vi "Actor Core.vi"(8 "error in":errorcluster, 11 "Chef Controller in":refnum<class "Chef Controller.lvclass">) -> (0 "error out":errorcluster, 3 "Actor out":refnum<class "Actor.lvclass">)   [LabVIEW 2024, in "Chef Controller.lvlib" / "Chef Controller.lvclass"]
doc: "<p>(<strong>Filename</strong>: <span class=\"dnl\">Actor Framework.lvlib:Actor.lvclass:Actor Core.vi</span>)</p>\n<p>Receives messages to the actor, reacts to them, and initiates any error handling that may shut the actor down.</p>\n<p>Descendant classes may override this VI to append parallel tasks for the actor to complete while it handles messages. Overrides use the <a href=\"nihelplauncher://docs/csh?context=lvcore_glang_udclass\">Call Parent Class Method</a> node.</p>"
uses:
  Chef Controller.lvclass
  Chef Controller.lvclass/Chef Controller.ctl
  <vilib>/ActorFramework/Actor/Actor.lvclass
  Chef View/Chef View.lvclass
  C:/Program Files/National Instruments/LabVIEW 2024/vi.lib/ActorFramework/Actor/Actor.lvclass
  G:/Leveling/LabVIEW/Learning/Actor Framework/chef/Chef View/Chef View.lvclass
  G:/Leveling/LabVIEW/Learning/Actor Framework/chef/Chef Controller/Chef Controller/Chef Controller.lvclass
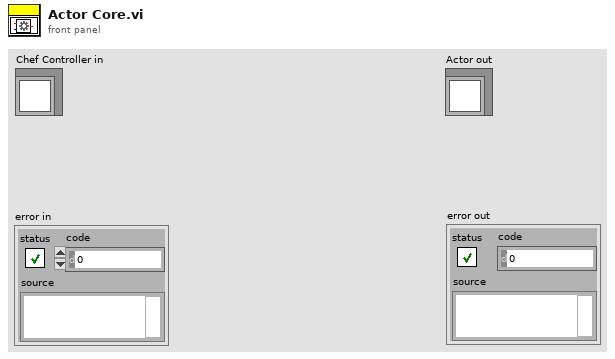
[diagram p1: front panel]
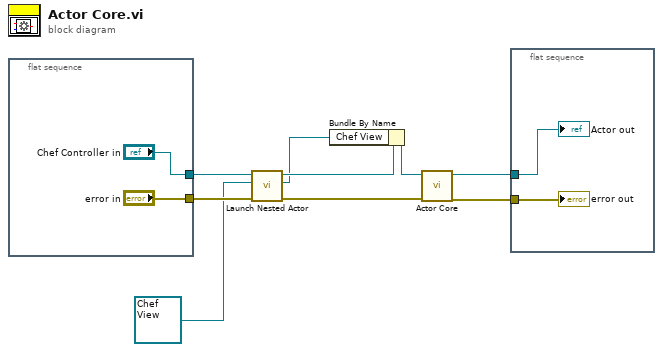
[diagram p0: block diagram]
diagram:
  n1 = flat-sequence {
    tunnel: ["error in"] -> w7
    tunnel: ["Chef Controller in"] -> w5
    frame #0 {
    }
  }
  n2 = call <vilib>:"Launch Nested Actor.vi"("error in (no error)"=w7, "Nested Actor"=refnum<class "Chef View.lvclass"> refnum ("Chef View.lvlib:Chef View.lvclass"), "Caller Actor in"=w5) -> ("error out"=w6:errorcluster, "Nested Actor's Enqueuer"=w1:refnum<class "Message Enqueuer.lvclass">, "Caller Actor out"=w4:refnum<class "Chef Controller.lvclass">)  [unwired: 6 in]
  n3 = Bundle By Name(cluster=w4, "Chef View"=w1) -> (w2:refnum<class "Chef Controller.lvclass">)
  n4 = call-parent "Actor Core.vi"("error in"=w6, "Actor in"=w2) -> ("error out"=w9:errorcluster, "Actor out"=w8:refnum<class "Actor.lvclass">)  [unwired: 8 in]
  n5 = flat-sequence {
    tunnel: w9 -> [w13]
    tunnel: w8 -> [w12]
    frame #0 {
      "error out" <- w13
      "Actor out" <- w12
    }
  }
